vi "ActorDatabase-PerformInsert.vi"(7 "Payload From Actor":string, 8 "error in (no error)":errorcluster, 11 "Database-Actor in":refnum<class "PartCertDatabase-Actor.lvclass">) -> (0 "error out":errorcluster, 3 "Database-Actor out":refnum<class "PartCertDatabase-Actor.lvclass">)   [LabVIEW 2013, in "PartCertDatabase-Actor.lvclass"]
uses:
  PartCertDatabase-Actor.lvclass
  PartCertDatabase-Actor.lvclass/PartCertDatabase-Actor.ctl
  ftw-dataflow/Core/src/Reflection/FTW-Reflection-Type.vi
  ftw-dataflow/Core/src/JSON/FTW-JSON-Core-LibraryFilepath.vi
  ftw-dataflow/Core/src/JSON/FTW-JSON-Core-GetFlattenedValue.vi
  ftw-dataflow/Core/src/JSON/FTW-JSON-Core-LibraryError.vi
  ftw-dataflow/Core/utils/CodeGen/JSON Deserialize/FTW-JSON-Deserialize.xnode
  Reuse Library/Database API/PartCertDatabase-API.lvclass
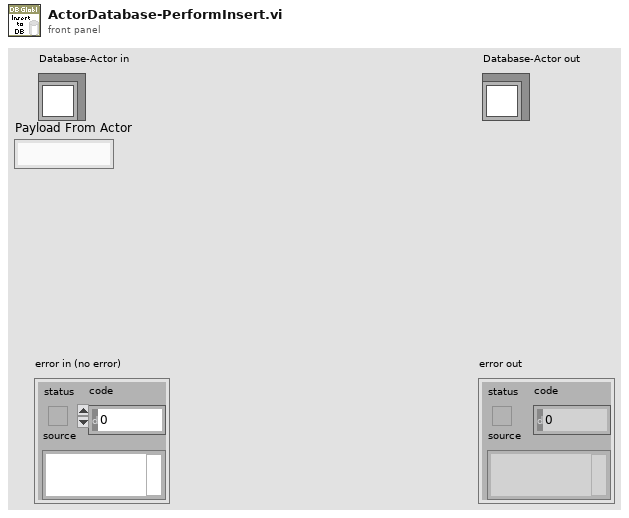
[diagram p1: front panel]
types:
  T1 = cluster{"New Inventory Assembled Part Number to Add":string, "On the Shelf":string, "Minimum":string, "Maximum":string}
  T2 = cluster{"Work Order":string, "Customer*":string, "Converted Start Date (String)":string, "Converted Due Date (String)":string, "Type Part Number*":string, "Part Number Description":string, "Quantity To Make":string, "Note - Special Instructions":string, "Assigned?":string, "Date Created":string, "Sales Order*":string, "Date Closed":string, "Status of Work Order":string, "Manufactured":string, "Inspected":string, "Approved":string, "Total Time to Manufacture":string, "Total Time to Inspect":string, "Path For PDF Special Instructions":string, "Reason For Closure":string, "RMA":string, "Manufacture User Notes":string, "Inspector User Notes":string, "Pull Inventory Note":string, "Stock Inventory Note":string}
  T3 = cluster{"Table":string, "SQL Statement":string, "Update All":bool, "Payload":string, "Reply Command":string, "Type Of Insertion":i32}
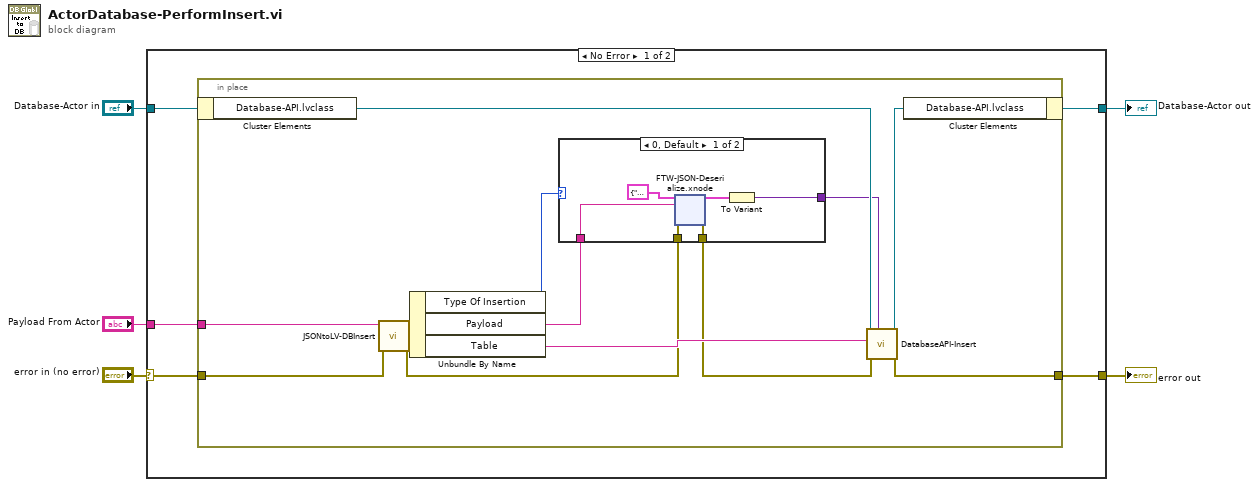
[diagram p0: block diagram]
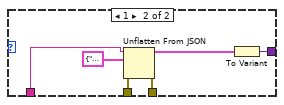
[diagram p2: hidden frame]
diagram:
  n1 = case shown="No Error" "error in (no error)" {
    selector: "error in (no error)" -> [w10 w70]
    tunnel: [w9 w70] -> w4
    tunnel: [w7 w69] -> w2
    tunnel: "Database-Actor in" -> [w8 w69]
    tunnel: "Payload From Actor" -> [w6 _]
    frame No Error {
      n2 = in-place {
        in-place-border: w10 -> [w20]
        in-place-border: [w19] -> w9
        in-place-border: w6 -> [w15]
        n3 = in-place-cluster #1(w8) -> ("Database-API.lvclass"=w17:refnum<class "PartCertDatabase-API.lvclass">)
        n4 = call "JSONtoLV-DBInsert.vi"("error in"=w20, "Output JSON Object"=w15) -> ("error out"=w13:errorcluster, "value"=w22:T3)  [unwired: 8 in]
        n5 = Unbundle By Name(w22) -> ("Type Of Insertion"=w18:i32, "Payload"=w14:string, "Table"=w21:string)
        n6 = case shown="0, Default" w18 {
          tunnel: w14 -> [w27 w66]
          tunnel: [w25 w68] -> w11
          tunnel: w13 -> [w24 w63]
          tunnel: [w23 w67] -> w12
          frame 0, Default {
            n7 = xnode "FTW-JSON-Deserialize.xnode"("Type and Defaults"=T1 {"New Inventory Assembled Part Number to Add"="", "On the Shelf"="", "Minimum"="", "Maximum"=""} ("cluster"), "JSON String"=w27, "error in"=w24) -> ("Values"=w26:T1, "error out"=w23:errorcluster)
            n8 = To Variant(anything=w26) -> (Variant=w25:variant)
          }
          frame 1 {
            n9 = Unflatten From JSON(JSON string=w66, type and defaults=T2 {"Work Order"="", "Customer*"="", "Converted Start Date (String)"="", "Converted Due Date (String)"="", "Type Part Number*"="", "Part Number Description"="", "Quantity To Make"="", "Note - Special Instructions"="", "Assigned?"="", "Date Created"="", "Sales Order*"="", "Date Closed"="", "Status of Work Order"="", "Manufactured"="", "Inspected"="", "Approved"="", "Total Time to Manufacture"="", "Total Time to Inspect"="", "Path For PDF Special Instructions"="", "Reason For Closure"="", "RMA"="", "Manufacture User Notes"="", "Inspector User Notes"="", "Pull Inventory Note"="", "Stock Inventory Note"=""} ("cluster"), error in (no error)=w63) -> (value=w64:T2, error out=w67:errorcluster)  [unwired: 4 in]
            n10 = To Variant(anything=w64) -> (Variant=w68:variant)
          }
        }
        n11 = call "DatabaseAPI-Insert.vi"("Cluster Data for DB"=w11, "error in (no error)"=w12, "Table"=w21, "Database-API in"=w17) -> ("error out"=w19:errorcluster, "Database-API out"=w16:refnum<class "PartCertDatabase-API.lvclass">)  [unwired: 6 in]
        n12 = in-place-cluster #1("Database-API.lvclass"=w16) -> (w7:refnum<class "PartCertDatabase-Actor.lvclass">)
      }
    }
    frame Error {
    }
  }
  "error out" <- w4
  "Database-Actor out" <- w2
